vi "Keithley_2400_source_meter.vi"() -> ()   [LabVIEW 2018]
uses:
  <vilib>/Analysis/baseanly.llb/Mean (DBL).vi
  <instrlib>/Keithley 24XX/Public/Data/Read (Multiple Points).vi
  <vilib>/Analysis/1siggen.llb/Ramp Pattern by Delta.vi
  <instrlib>/Keithley 24XX/Keithley 24XX.lvlib
  <vilib>/Analysis/NI_AALBase.lvlib
panel:
  out "Over Load":bool
  in  "Grid":enum32{"Radio Selection 1", "Radio Selection 2"}(radio)=enum."Radio Selection 2"
  in  "Save":bool=TRUE
  in  "File Name":string="Name"
  out "Current [A]":dbl format="%0.6e"
  out "Resistance [ohm]":dbl format="%0.6e"
  out "Resistance":cluster{dbl, "mean":dbl}[](graph) caption="Processed X-Rey Plot"
  out "Current":cluster{dbl, "mean":dbl}[](graph) caption="Processed X-Rey Plot"
  in  "Setup":T1={"Current Manual Range"=1.0, "Current Auto Range "=TRUE, "Comunication Port"="COM8", "Compliance  Level"=0.1, "Fixed Voltage"=0.5, "Source Mode"=0, "stop"=FALSE, "Sweep"=FALSE, "start"=0.0, "stop [V]"=0.8, "step"=0.01, "Progress"=0, "Current Limit [A]"=0.002, "Resistance Manual Range"=1.0, "direction"=FALSE} {"Current Limit [A]" format="%#_6e"; "Progress" scale=0.0..100.0; "Source Mode" items=["Voltage", "Current"]}
  # "%"
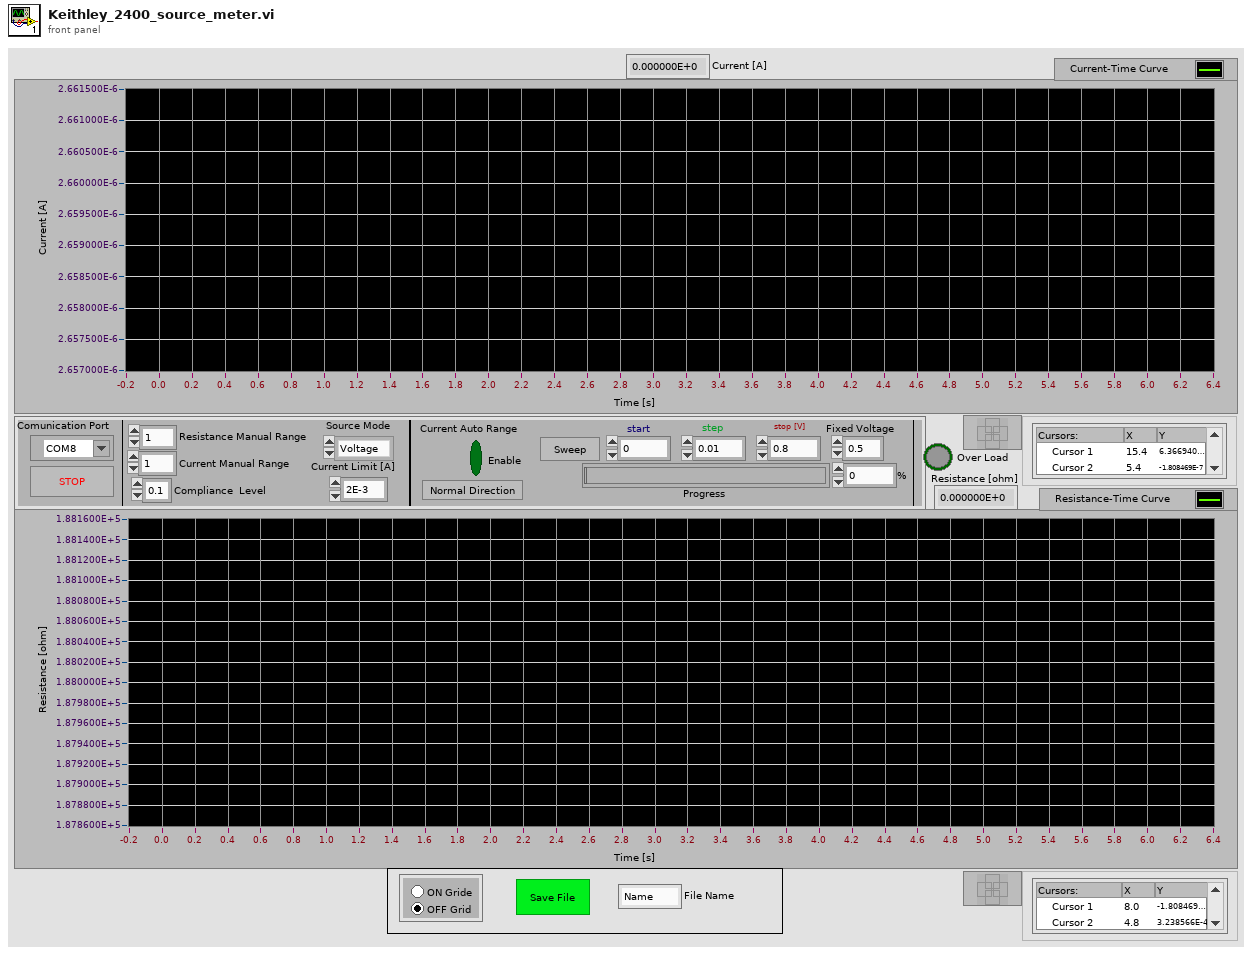
[diagram p1: front panel]
types:
  T1 = cluster{"Current Manual Range":dbl, "Current Auto Range ":bool, "Comunication Port":refnum<visa-resource-name>, "Compliance  Level":dbl, "Fixed Voltage":dbl, "Source Mode":u16, "stop":bool, "Sweep":bool, "start":dbl, "stop [V]":dbl, "step":dbl, "Progress":u8, "Current Limit [A]":dbl, "Resistance Manual Range":dbl, "direction":bool}
  T2 = cluster{"Baud Rate":u32, "Parity":u16, "Data Bits":u16, "Stop Bits":u16, "Flow Control":u16}
  T3 = enum16{"open", "replace", "create", "open or create", "replace or create", "replace or create with confirmation"}
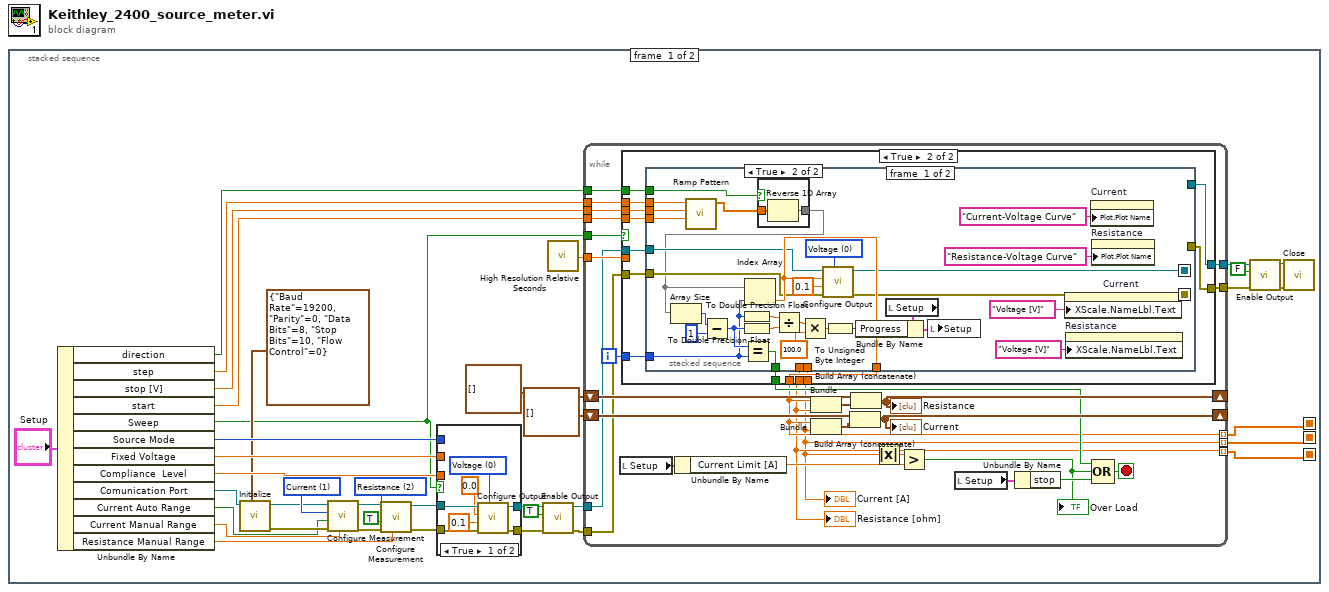
[diagram p0: block diagram]
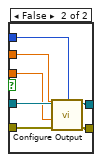
[diagram p2: hidden frame]
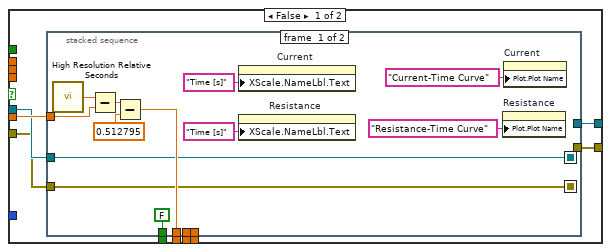
[diagram p3: hidden frame]
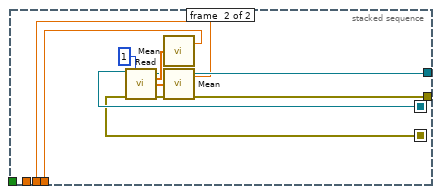
[diagram p4: hidden frame]
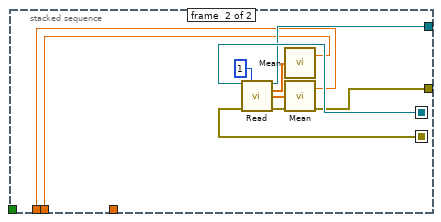
[diagram p6: hidden frame]
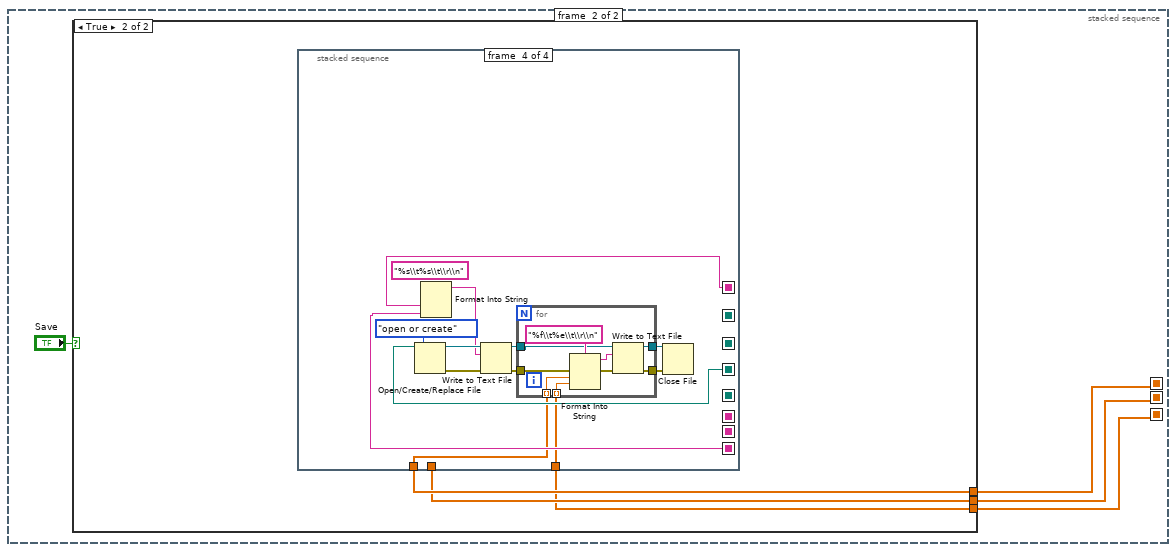
[diagram p7: hidden frame]
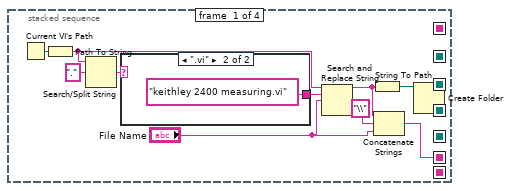
[diagram p9: hidden frame]
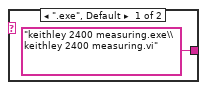
[diagram p10: hidden frame]
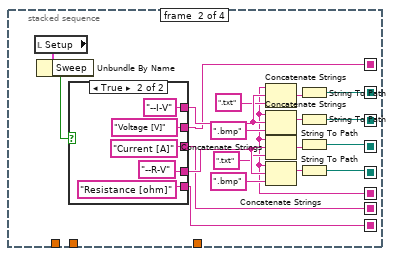
[diagram p11: hidden frame]
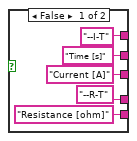
[diagram p12: hidden frame]
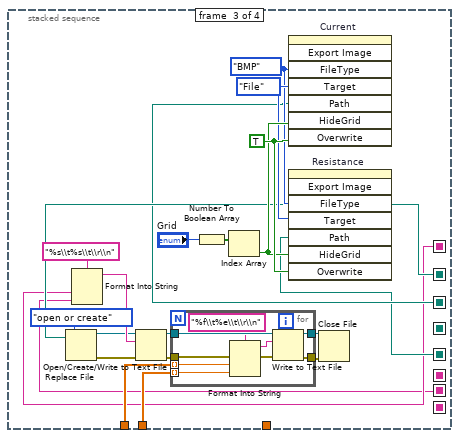
[diagram p13: hidden frame]
diagram:
  n1 = stacked-sequence {
    seq-local: [w3 _] -> [_ w169]
    seq-local: [w1 _] -> [_ w167]
    seq-local: [w2 _] -> [_ w168]
    frame #0 {
      w10 = u16 2 items=["Volts", "Current", "Resistance"] ("Function (0: Volts)")
      w39 = u16 1 items=["Volts", "Current", "Resistance"] ("Function (0: Volts)")
      n2 = Unbundle By Name("Setup") -> ("direction"=w4:bool, "step"=w21:dbl, "stop [V]"=w20:dbl, "start"=w19:dbl, "Sweep"=w16:bool, "Source Mode"=w25:u16, "Fixed Voltage"=w26:dbl, "Compliance  Level"=w27:dbl, "Comunication Port"=w28:refnum<visa-resource-name>, "Current Auto Range"=w24:bool, "Current Manual Range"=w8:dbl, "Resistance Manual Range"=w9:dbl)
      n3 = call <instrlib>:"Initialize.vi"("Serial Configuration"=T2 {"Baud Rate"=19200, "Parity"=0, "Data Bits"=8, "Stop Bits"=10, "Flow Control"=0}, "VISA resource name"=w28) -> ("error out"=w37:errorcluster, "VISA resource name out"=w38:refnum<visa-resource-name>)  [unwired: 8 in]
      n4 = call <instrlib>:"Configure Measurement.vi"("Manual Range (1.0)"=w8, "error in (no error)"=w37, "Enable Auto Range (T:Enable)"=w24, "Function (0: Volts)"=w39, "VISA resource name"=w38) -> ("error out"=w11:errorcluster, "VISA resource name out"=w14:refnum<visa-resource-name>)  [unwired: 5 in]
      n5 = call <instrlib>:"Configure Measurement.vi"("Manual Range (1.0)"=w9, "error in (no error)"=w11, "Enable Auto Range (T:Enable)"=TRUE, "Function (0: Volts)"=w10, "VISA resource name"=w14) -> ("error out"=w12:errorcluster, "VISA resource name out"=w13:refnum<visa-resource-name>)  [unwired: 5 in]
      n6 = case shown="True" w16 {
        tunnel: w12 -> [w44 w53]
        tunnel: w13 -> [w43 w52]
        tunnel: [w46 w51] -> w31
        tunnel: [w45 w50] -> w30
        tunnel: w27 -> [_ w49]
        tunnel: w26 -> [_ w48]
        tunnel: w25 -> [_ w47]
        frame True {
          w40 = u16 0 items=["Voltage", "Current"] ("Source Mode  (0: Voltage)")
          n7 = call <instrlib>:"Configure Output.vi"("Source Mode  (0: Voltage)"=w40, "error in (no error)"=w44, "Compliance  Level (0.1)"=0.1, "Output Level (0)"=0.0, "VISA resource name"=w43) -> ("error out"=w45:errorcluster, "VISA resource name out"=w46:refnum<visa-resource-name>)  [unwired: 5 in]
        }
        frame False {
          n8 = call <instrlib>:"Configure Output.vi"("Source Mode  (0: Voltage)"=w47, "error in (no error)"=w53, "Compliance  Level (0.1)"=w49, "Output Level (0)"=w48, "VISA resource name"=w52) -> ("error out"=w50:errorcluster, "VISA resource name out"=w51:refnum<visa-resource-name>)  [unwired: 5 in]
        }
      }
      n9 = call <instrlib>:"Enable Output.vi"("error in (no error)"=w30, "Enable Output (T: Enable)"=TRUE, "VISA resource name"=w31) -> ("error out"=w35:errorcluster, "VISA resource name out"=w34:refnum<visa-resource-name>)  [unwired: 7 in]
      n10 = call <vilib>:"High Resolution Relative Seconds.vi"() -> ("relative seconds"=w15:dbl)
      n11 = while {
        shift-right: [w78] -> _
        shift-left: cluster{dbl, "mean":dbl}[] [] -> [w80]
        shift-right: [w77] -> _
        shift-left: cluster{dbl, "mean":dbl}[] [] -> [w75]
        tunnel: w21 -> [w74]
        tunnel: w20 -> [w73]
        tunnel: w19 -> [w72]
        tunnel: w16 -> [w66]
        tunnel: w15 -> [w62]
        tunnel: w34 -> [w60]
        tunnel: w35 -> [w59]
        tunnel: [w61] -> w3 mode=indexing
        tunnel: [w55] -> w2 mode=indexing
        tunnel: [w56] -> w1 mode=indexing
        tunnel: [w58] -> w6
        tunnel: [w57] -> w5
        tunnel: w4 -> [w54]
        i -> [w63]
        stop <- w70 stop-if-true
        n12 = local read "Setup"() -> (w68:T1)
        n13 = case shown="True" w66 {
          tunnel: w74 -> [_ w124]
          tunnel: w73 -> [_ w123]
          tunnel: w72 -> [_ w122]
          tunnel: [w90 w121] -> w69
          tunnel: w63 -> [_ w120]
          tunnel: w62 -> [w89 _]
          tunnel: [w88 w115] -> w61
          tunnel: w60 -> [w87 w119]
          tunnel: w59 -> [w86 w118]
          tunnel: [w85 w117] -> w58
          tunnel: [w84 w116] -> w57
          tunnel: [w83 w113] -> w55
          tunnel: [w82 w114] -> w56
          tunnel: w54 -> [_ w112]
          frame False {
            n14 = stacked-sequence {
              seq-local: [w91 _] -> [_ w106]
              seq-local: [w92 _] -> [_ w105]
              tunnel: [FALSE _] -> w90
              tunnel: w89 -> [w98 _]
              tunnel: [w97 _] -> w88
              tunnel: w87 -> [w91 _]
              tunnel: w86 -> [w92 _]
              tunnel: [_ w108] -> w85
              tunnel: [_ w107] -> w84
              tunnel: [_ w104] -> w83
              tunnel: [_ w103] -> w82
              frame #0 {
                n15 = call <vilib>:"High Resolution Relative Seconds.vi"() -> ("relative seconds"=w100:dbl)
                n16 = Subtract(x=w100, y=w98) -> (x-y=w101:dbl)
                n17 = Subtract(x=w101, y=0.512795) -> (x-y=w97:dbl)
                n18 = property on="Current" class="XYGraph (strict)"("XScale.NameLbl.Text"="Time [s]" ("X Scale.Name Label.Text")) -> ()  [unwired: 2 in, 2 out]
                n19 = property on="Resistance" class="XYGraph (strict)"("XScale.NameLbl.Text"="Time [s]" ("X Scale.Name Label.Text")) -> ()  [unwired: 2 in, 2 out]
                n20 = property on="Resistance" class="XYGraph (strict)"("Plot.Plot Name"="Resistance-Time Curve") -> ()  [unwired: 2 in, 2 out]
                n21 = property on="Current" class="XYGraph (strict)"("Plot.Plot Name"="Current-Time Curve") -> ()  [unwired: 2 in, 2 out]
              }
              frame #1 {
                n22 = call-poly <instrlib>:"Read.vi"("VISA resource name"=w106, "Sample Count (1)"=1, "error in (no error)"=w105) -> ("VISA resource name out"=w108:refnum<visa-resource-name>, "Current"=w110:sgl[], "Resistance"=w111:sgl[], "error out"=w107:errorcluster)  [unwired: 6 in, 3 out]
                n23 = call-poly <vilib>:"Mean.vi"("X"=w110) -> ("mean"=w104:dbl)  [unwired: 1 out]
                n24 = call-poly <vilib>:"Mean.vi"("X"=w111) -> ("mean"=w103:dbl)  [unwired: 1 out]
              }
            }
          }
          frame True {
            n25 = stacked-sequence {
              seq-local: [w129 _] -> [_ w163]
              seq-local: [w128 _] -> [_ w162]
              tunnel: w124 -> [w143 _]
              tunnel: w123 -> [w142 _]
              tunnel: w122 -> [w141 _]
              tunnel: [w140 _] -> w121
              tunnel: w120 -> [w137 _]
              tunnel: [w136 _] -> w115
              tunnel: w119 -> [w131 _]
              tunnel: w118 -> [w130 _]
              tunnel: [_ w161] -> w117
              tunnel: [_ w160] -> w116
              tunnel: [_ w159] -> w114
              tunnel: [_ w158] -> w113
              tunnel: w112 -> [w126 _]
              frame #0 {
                w138 = u16 0 items=["Voltage", "Current"] ("Source Mode  (0: Voltage)")
                n26 = call-poly <vilib>:"Ramp Pattern.vi"("start"=w141, "end"=w142, "delta"=w143) -> ("Ramp Pattern"=w127:dbl[])  [unwired: 6 in, 2 out]
                n27 = To Double Precision Float(number=w137) -> (double precision float=w149:dbl)
                n28 = case shown="True" w126 {
                  tunnel: w127 -> [w155 w157]
                  tunnel: [w155 w156] -> w125
                  frame False {
                  }
                  frame True {
                    n29 = Reverse 1D Array(array=w157) -> (reversed array=w156:dbl[])
                  }
                }
                n30 = Array Size(array=w125) -> (size(s)=w151:i32)
                n31 = Subtract(x=w151, y=1) -> (x-y=w150:i32)
                n32 = To Double Precision Float(number=w150) -> (double precision float=w147:dbl)
                n33 = Equal?(x=w150, y=w137) -> (x = y?=w140:bool)
                n34 = Index Array(array=w125, index=w137) -> (element=w136:dbl)
                n35 = Divide(x=w149, y=w147) -> (x/y=w146:dbl)
                n36 = Multiply(x=w146, y=100.0) -> (x*y=w148:dbl)
                n37 = call <instrlib>:"Configure Output.vi"("Source Mode  (0: Voltage)"=w138, "error in (no error)"=w130, "Compliance  Level (0.1)"=0.1, "Output Level (0)"=w136, "VISA resource name"=w131) -> ("error out"=w128:errorcluster, "VISA resource name out"=w129:refnum<visa-resource-name>)  [unwired: 5 in]
                n38 = To Unsigned Byte Integer(number=w148) -> (unsigned 8bit integer=w154:u8)
                n39 = local read "Setup"() -> (w152:T1)
                n40 = Bundle By Name(cluster=w152, "Progress"=w154) -> (w153:T1)
                n41 = local write "Setup"(w153) -> ()
                n42 = property on="Current" class="XYGraph (strict)"("XScale.NameLbl.Text"="Voltage [V]" ("X Scale.Name Label.Text")) -> ()  [unwired: 2 in, 2 out]
                n43 = property on="Resistance" class="XYGraph (strict)"("XScale.NameLbl.Text"="Voltage [V]" ("X Scale.Name Label.Text")) -> ()  [unwired: 2 in, 2 out]
                n44 = property on="Current" class="XYGraph (strict)"("Plot.Plot Name"="Current-Voltage Curve") -> ()  [unwired: 2 in, 2 out]
                n45 = property on="Resistance" class="XYGraph (strict)"("Plot.Plot Name"="Resistance-Voltage Curve") -> ()  [unwired: 2 in, 2 out]
              }
              frame #1 {
                n46 = call-poly <instrlib>:"Read.vi"("VISA resource name"=w163, "Sample Count (1)"=1, "error in (no error)"=w162) -> ("VISA resource name out"=w161:refnum<visa-resource-name>, "Current"=w165:sgl[], "Resistance"=w166:sgl[], "error out"=w160:errorcluster)  [unwired: 6 in, 3 out]
                n47 = call-poly <vilib>:"Mean.vi"("X"=w165) -> ("mean"=w158:dbl)  [unwired: 1 out]
                n48 = call-poly <vilib>:"Mean.vi"("X"=w166) -> ("mean"=w159:dbl)  [unwired: 1 out]
              }
            }
          }
        }
        "Resistance [ohm]" <- w56
        "Current [A]" <- w55
        n49 = Unbundle By Name(w68) -> ("Current Limit [A]"=w67:dbl)
        n50 = Bundle(w61, "mean"=w56) -> (w76:cluster{dbl, "mean":dbl})  [unwired: 1 in]
        n51 = Bundle(w61, "mean"=w55) -> (w81:cluster{dbl, "mean":dbl})  [unwired: 1 in]
        n52 = Build Array (concatenate)(w80, w81) -> (w78:cluster{dbl, "mean":dbl}[])
        "Current" <- w78
        n53 = Build Array (concatenate)(w75, w76) -> (w77:cluster{dbl, "mean":dbl}[])
        "Resistance" <- w77
        n54 = Absolute Value(x=w55) -> (abs(x)=w71:dbl)
        n55 = Greater?(x=w71, y=w67) -> (0:w64:bool)
        "Over Load" <- w64
        n56 = local read "Setup"() -> (w79:T1)
        n57 = Unbundle By Name(w79) -> ("stop"=w65:bool)
        n58 = Compound Arithmetic op=OR(w69, w64, w65) -> (w70:bool)
      }
      n59 = call <instrlib>:"Enable Output.vi"("error in (no error)"=w5, "Enable Output (T: Enable)"=FALSE, "VISA resource name"=w6) -> ("error out"=w17:errorcluster, "VISA resource name out"=w18:refnum<visa-resource-name>)  [unwired: 7 in]
      n60 = call <instrlib>:"Close.vi"("error in (no error)"=w17, "VISA resource name"=w18) -> ()  [unwired: 9 in, 1 out]
    }
    frame #1 {
      n61 = case shown="True" "Save" {
        tunnel: w169 -> [_ w173]
        tunnel: w168 -> [_ w172]
        tunnel: w167 -> [_ w171]
        frame False {
        }
        frame True {
          n62 = stacked-sequence {
            seq-local: [w174 _ _ _] -> [_ w193 _ _]
            seq-local: [_ w190 _ _] -> [_ _ _ w249]
            seq-local: [_ w191 _ _] -> [_ _ w216 _]
            seq-local: [_ w192 _ _] -> [_ _ w217 w250]
            seq-local: [_ w186 _ _] -> [_ _ w222 _]
            seq-local: [_ w187 _ _] -> [_ _ w221 _]
            seq-local: [_ w188 _ _] -> [_ _ _ w251]
            seq-local: [_ w189 _ _] -> [_ _ w220 _]
            tunnel: w173 -> [_ _ w219 w248]
            tunnel: w172 -> [_ _ w218 _]
            tunnel: w171 -> [_ _ _ w247]
            frame #0 {
              n63 = Current VI's Path() -> (path=w178:path)
              n64 = Path To String(path=w178) -> (string=w183:string)
              n65 = Search/Split String(string=w183, search string/char (-)=".") -> (match + rest of string=w177:string)  [unwired: 1 in, 2 out]
              n66 = case shown="\".vi\"" w177 {
                tunnel: ["keithley 2400 measuring.exe\\keithley 2400 measuring.vi" ("regular expression") "keithley 2400 measuring.vi" ("regular expression")] -> w176
                frame ".exe", Default {
                }
                frame ".vi" {
                }
              }
              n67 = Search and Replace String(input string=w183, search string=w176, replace string="File Name") -> (result string=w180:string)  [unwired: 5 in, 3 out]
              n68 = String To Path(string=w180) -> (path=w179:path)
              n69 = Concatenate Strings(w180, "\\" ("string"), "File Name") -> (w174:string)
              n70 = Create Folder(path (use dialog)=w179) -> ()  [unwired: 2 in, 3 out]
            }
            frame #1 {
              n71 = local read "Setup"() -> (w202:T1)
              n72 = Unbundle By Name(w202) -> ("Sweep"=w203:bool)
              n73 = case shown="True" w203 {
                tunnel: ["--I-T" ("string") "--I-V" ("string")] -> w204
                tunnel: ["--R-T" ("string") "--R-V" ("string")] -> w205
                tunnel: ["Time [s]" ("Signal Name") "Voltage [V]" ("Signal Name")] -> w192
                tunnel: ["Resistance [ohm]" ("Signal Name") "Resistance [ohm]" ("Signal Name")] -> w190
                tunnel: ["Current [A]" ("Signal Name") "Current [A]" ("Signal Name")] -> w191
                frame False {
                }
                frame True {
                }
              }
              n74 = Concatenate Strings(w193, w204, ".txt" ("string")) -> (w195:string)
              n75 = Concatenate Strings(w193, w204, ".bmp" ("string")) -> (w194:string)
              n76 = Concatenate Strings(w193, w205, ".txt" ("string")) -> (w196:string)
              n77 = Concatenate Strings(w193, w205, ".bmp" ("string")) -> (w197:string)
              n78 = String To Path(string=w195) -> (path=w186:path)
              n79 = String To Path(string=w194) -> (path=w187:path)
              n80 = String To Path(string=w196) -> (path=w188:path)
              n81 = String To Path(string=w197) -> (path=w189:path)
            }
            frame #2 {
              w224 = enum32{"BMP", "EPS", "EMF", "PICT"}."BMP" ("File Type")
              w227 = TRUE ("Always Overwrite")
              w225 = enum32{"File", "Clipboard"}."File" ("Target")
              n82 = Open/Create/Replace File(file path (use dialog)=w222, operation (0:open)=T3."open or create") -> (refnum out=w235:refnum<file>, error out=w236:errorcluster)  [unwired: 4 in, 1 out]
              n83 = Format Into String(format string="%s\\t%s\\t\\r\\n", w217, w216) -> (resulting string=w237:string)  [unwired: 2 in, 1 out]
              n84 = Write to Text File(file (use dialog)=w235, text=w237, error in=w236) -> (refnum out=w234:refnum<file>, error out=w233:errorcluster)  [unwired: 1 in, 1 out]
              n85 = for {
                tunnel: w234 -> [w243]
                tunnel: [w245] -> w230
                tunnel: w233 -> [w240]
                tunnel: [w244] -> w231
                tunnel: w219 -> [w239] mode=indexing
                tunnel: w218 -> [w238] mode=indexing
                n86 = Format Into String(format string="%f\\t%e\\t\\r\\n", error in=w240, w239, w238) -> (resulting string=w246:string, error out=w241:errorcluster)  [unwired: 1 in]
                n87 = Write to Text File(file (use dialog)=w243, text=w246, error in=w241) -> (refnum out=w245:refnum<file>, error out=w244:errorcluster)  [unwired: 1 in, 1 out]
              }
              n88 = Number To Boolean Array(number="Grid") -> (Boolean array=w223:bool[])
              n89 = Index Array(array=w223) -> (element=w226:bool)  [unwired: 1 in]
              n90 = invoke on="Current" class="XYGraph (strict)" method="Export Image"("FileType"=w224, "Target"=w225, "Path"=w221, "HideGrid"=w226, "Overwrite"=w227) -> ()  [unwired: 3 in, 8 out]
              n91 = invoke on="Resistance" class="XYGraph (strict)" method="Export Image"("FileType"=w224, "Target"=w225, "Path"=w220, "HideGrid"=w226, "Overwrite"=w227) -> ()  [unwired: 3 in, 8 out]
              n92 = Close File(refnum=w230, error in=w231) -> ()  [unwired: 2 out]
            }
            frame #3 {
              (unwired) "%s\\t%s\\t\\r\\n" ("format string")
              n93 = Open/Create/Replace File(file path (use dialog)=w251, operation (0:open)=T3."open or create") -> (refnum out=w254:refnum<file>, error out=w253:errorcluster)  [unwired: 4 in, 1 out]
              n94 = Format Into String(w250, w249) -> (resulting string=w252:string)  [unwired: 3 in, 1 out]
              n95 = Write to Text File(file (use dialog)=w254, text=w252, error in=w253) -> (refnum out=w257:refnum<file>, error out=w256:errorcluster)  [unwired: 1 in, 1 out]
              n96 = for {
                tunnel: w256 -> [w264]
                tunnel: w257 -> [w265]
                tunnel: [w263] -> w258
                tunnel: [w262] -> w259
                tunnel: w248 -> [w261] mode=indexing
                tunnel: w247 -> [w260] mode=indexing
                n97 = Format Into String(format string="%f\\t%e\\t\\r\\n", error in=w264, w261, w260) -> (resulting string=w266:string, error out=w268:errorcluster)  [unwired: 1 in]
                n98 = Write to Text File(file (use dialog)=w265, text=w266, error in=w268) -> (refnum out=w262:refnum<file>, error out=w263:errorcluster)  [unwired: 1 in, 1 out]
              }
              n99 = Close File(refnum=w259, error in=w258) -> ()  [unwired: 2 out]
            }
          }
        }
      }
    }
  }
